vi "File Save Result.vi"(4 "TDMs?":bool, 6 "wfm Info":T1(array[cluster]), 7 "file path":path caption="file path (dialog if empty)", 8 "error in":errorcluster caption="错误输入（无错误）", 9 "wfm name":string[](array[string]), 10 "WFM Out":waveform(dbl)[](array[waveform]), 11 "Compute Result":string[][](array[string])) -> (0 "error out":errorcluster caption="错误输出")   [LabVIEW 2012]
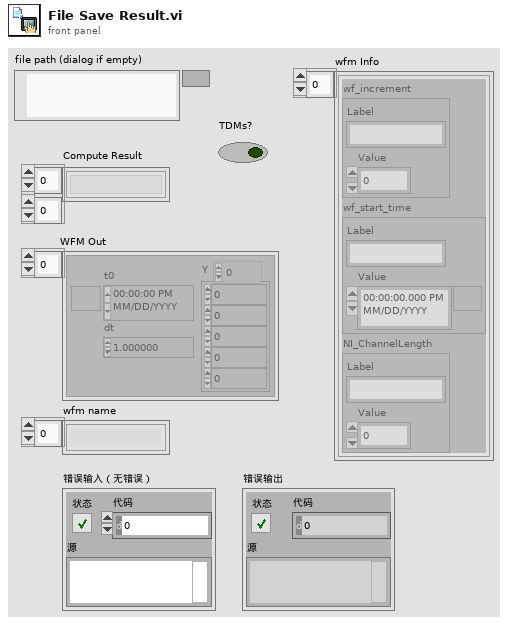
[diagram p1: front panel]
types:
  T1 = cluster{"wf_increment":cluster{"Label":string, "Value":dbl}, "wf_start_time":cluster{"Label":string, "Value":timestamp}, "NI_ChannelLength":cluster{"Label":string, "Value":dbl}}[]
  T2 = enum16{"open", "replace", "create", "open or create", "replace or create", "replace or create with confirmation"}
  T3 = enum16{"open", "open or create", "create or replace", "create", "open (read-only)"}
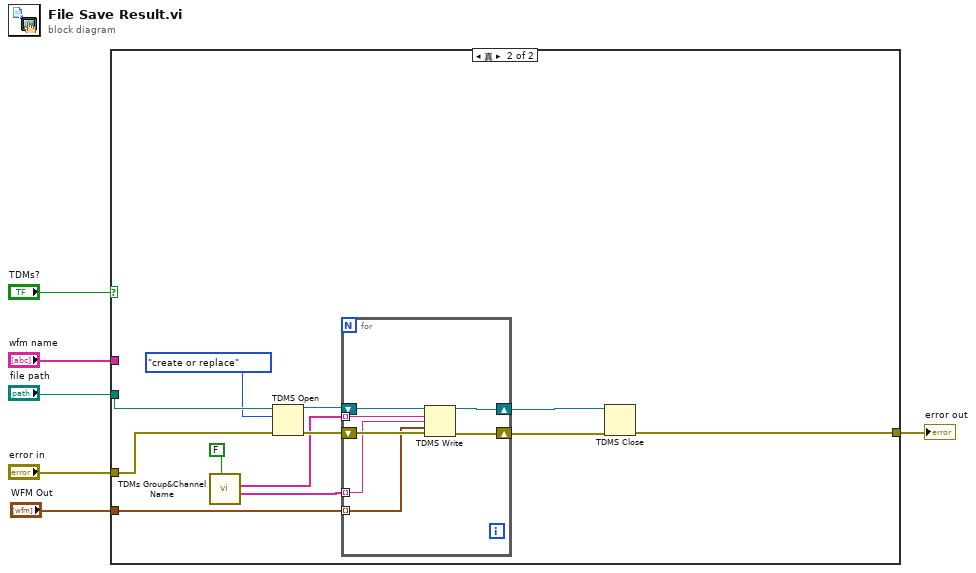
[diagram p0: block diagram]
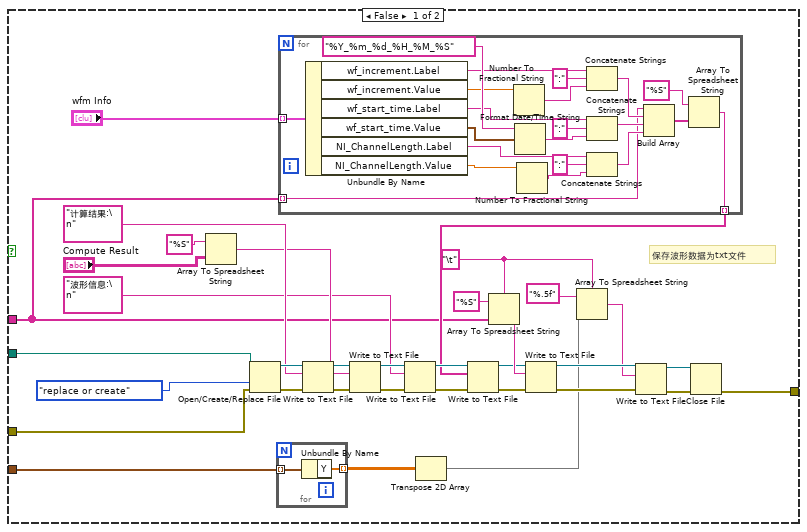
[diagram p2: hidden frame]
diagram:
  n1 = case shown="真" "TDMs?" {
    tunnel: "error in" -> [w29 w74]
    tunnel: [w28 w71] -> w5
    tunnel: "file path" -> [w9 w75]
    tunnel: "wfm name" -> [w8 _]
    tunnel: "WFM Out" -> [w7 w65]
    frame False {
      w36 = "\t" ("delimiter (\\t)")
      # "保存波形数据为txt文件"
      n2 = Array To Spreadsheet String(array="Compute Result", 3:"%S" ("格式字符串")) -> (spreadsheet string=w20:string)  [unwired: 1 in]
      n3 = Open/Create/Replace File(file path (use dialog)=w9, error in=w29, operation (0:open)=T2."replace or create" ("操作(0:open)")) -> (refnum out=w26:refnum<file>, error out=w27:errorcluster)  [unwired: 3 in, 1 out]
      n4 = for {
        tunnel: w7 -> [w63] mode=indexing
        tunnel: [w62] -> w33 mode=indexing
        n5 = Unbundle By Name(w63) -> ("Y"=w62:dbl[])
      }
      n6 = for {
        tunnel: "wfm Info" -> [w61] mode=indexing
        tunnel: w8 -> [w44] mode=indexing
        tunnel: [w41] -> w12 mode=indexing
        n7 = Unbundle By Name(w61) -> ("wf_increment.Label"=w57:string, "wf_increment.Value"=w58:dbl, "wf_start_time.Label"=w53:string, "wf_start_time.Value"=w60:timestamp, "NI_ChannelLength.Label"=w50:string, "NI_ChannelLength.Value"=w49:dbl)
        n8 = Number To Fractional String(number=w58) -> (F-format string=w55:string)  [unwired: 3 in]
        n9 = Format Date/Time String(time format string (%c)="%Y_%m_%d_%H_%M_%S" ("时间格式字符串(%c)"), seconds (now)=w60) -> (date/time string=w52:string)  [unwired: 1 in]
        n10 = Number To Fractional String(number=w49) -> (F-format string=w48:string)  [unwired: 3 in]
        n11 = Concatenate Strings(w57, ":" ("字符串"), w55) -> (w47:string)
        n12 = Concatenate Strings(w53, ":" ("字符串"), w52) -> (w46:string)
        n13 = Concatenate Strings(w50, ":" ("字符串"), w48) -> (w45:string)
        n14 = Build Array(w44, w47, w46, w45) -> (w43:string[])
        n15 = Array To Spreadsheet String(array=w43, 3:"%S" ("格式字符串")) -> (spreadsheet string=w41:string)  [unwired: 1 in]
      }
      n16 = Write to Text File(file (use dialog)=w26, text="计算结果:\n", error in=w27) -> (refnum out=w22:refnum<file>, error out=w21:errorcluster)  [unwired: 1 in, 1 out]
      n17 = Write to Text File(file (use dialog)=w22, text=w20, error in=w21) -> (refnum out=w19:refnum<file>, error out=w18:errorcluster)  [unwired: 1 in, 1 out]
      n18 = Write to Text File(file (use dialog)=w19, text="波形信息:\n", error in=w18) -> (refnum out=w17:refnum<file>, error out=w15:errorcluster)  [unwired: 1 in, 1 out]
      n19 = Transpose 2D Array(2D array=w33) -> (transposed array=w30:dbl[][])
      n20 = Write to Text File(file (use dialog)=w17, text=w12, error in=w15) -> (refnum out=w16:refnum<file>, error out=w14:errorcluster)  [unwired: 1 in, 1 out]
      n21 = Array To Spreadsheet String(delimiter (Tab)=w36, array=w8, 3:"%S" ("格式字符串")) -> (spreadsheet string=w37:string)
      n22 = Write to Text File(file (use dialog)=w16, text=w37, error in=w14) -> (refnum out=w38:refnum<file>, error out=w31:errorcluster)  [unwired: 1 in, 1 out]
      n23 = Array To Spreadsheet String(delimiter (Tab)=w36, array=w30, 3:"%.5f" ("format (%.3f)")) -> (spreadsheet string=w32:string)
      n24 = Write to Text File(file (use dialog)=w38, text=w32, error in=w31) -> (refnum out=w40:refnum<file>, error out=w39:errorcluster)  [unwired: 1 in, 1 out]
      n25 = Close File(refnum=w40, error in=w39) -> (error out=w28:errorcluster)  [unwired: 1 out]
    }
    frame True {
      n26 = call "TDMs Group&Channel Name.vi"("Ini?"=FALSE) -> ("Channel"=w68:string[], "Group"=w69:string[])  [unwired: 8 in, 1 out]
      n27 = TDMS Open(8:w74, 10:T3."create or replace" ("操作(0:open)"), 11:w75) -> (0:w73:errorcluster, 3:w67:refnum<k34>)  [unwired: 3 in]
      n28 = for {
        tunnel: w69 -> [w80] mode=indexing
        tunnel: w68 -> [w77] mode=indexing
        shift-right: [w81] -> w72
        shift-left: w73 -> [w82]
        shift-right: [w78] -> w66
        shift-left: w67 -> [w79]
        tunnel: w65 -> [w76] mode=indexing
        n29 = TDMS Write(0:w79, 5:w80, 7:w77, 9:w76, 11:w82) -> (4:w78:refnum<k34>, 15:w81:errorcluster)  [unwired: 1 in, 2 out]
      }
      n30 = TDMS Close(8:w72, 11:w66) -> (0:w71:errorcluster)  [unwired: 1 out]
    }
  }
  "error out" <- w5
